vi "GetCallerVIifInvalid.vi"(8 "error in (no error)":errorcluster, 11 "VI in":refnum<vi>) -> (0 "error out":errorcluster, 2 "Caller VI?":bool, 3 "VI out":refnum<vi>)   [LabVIEW 2014, in "RefManager(dev).lvlib"]
uses:
  RefManager(dev).lvlib
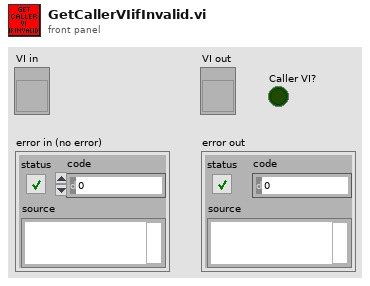
[diagram p1: front panel]
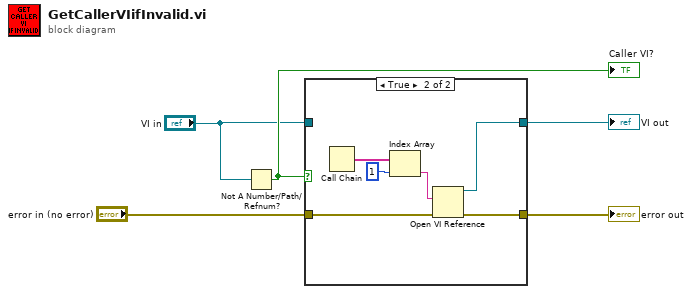
[diagram p0: block diagram]
diagram:
  n1 = Not A Number/Path/Refnum?(number/path/refnum="VI in") -> (NaN/Path/Refnum?=w3:bool)
  "Caller VI?" <- w3
  n2 = case shown="True" w3 {
    tunnel: [w7 w13] -> w5
    tunnel: "error in (no error)" -> [w7 w12]
    tunnel: [w6 w11] -> w1
    tunnel: "VI in" -> [w6 _]
    frame False {
    }
    frame True {
      n3 = Call Chain() -> (call chain=w8:string[])
      n4 = Index Array(array=w8, index=1) -> (element=w9:string)
      n5 = Open VI Reference(vi path=w9, error in (no error)=w12) -> (vi reference=w11:refnum<vi>, error out=w13:errorcluster)  [unwired: 4 in]
    }
  }
  "error out" <- w5
  "VI out" <- w1
